vi "flat_Secuence_bloqueo.vi"() -> ()   [LabVIEW 2020]
panel:
  out "Thermometer 4":u8(slide) scale=0.0..100.0
  out "Thermometer 3":u8(slide) scale=0.0..100.0
  out "Thermometer 2":u8(slide) scale=0.0..100.0
  out "Thermometer":u8(slide) scale=0.0..100.0
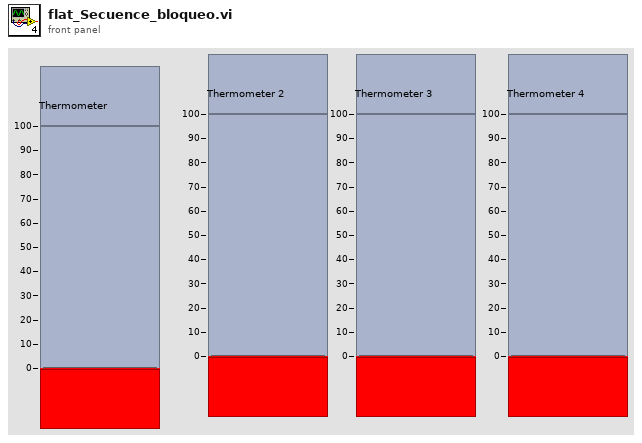
[diagram p1: front panel]
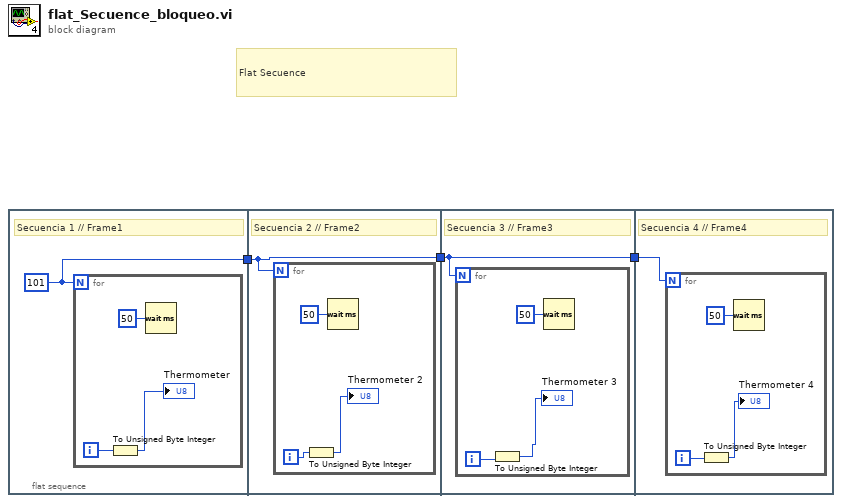
[diagram p0: block diagram]
diagram:
  # "Flat Secuence"
  n1 = flat-sequence {
    tunnel: [w4] -> w3
    tunnel: w3 -> [w8]
    tunnel: [w8] -> w2
    tunnel: w2 -> [w12]
    tunnel: [w12] -> w1
    tunnel: w1 -> [w16]
    frame #0 {
      w4 = 101
      # "Secuencia 1 // Frame1"
      n2 = for {
        N: w4 -> [_]
        i -> [w6]
        n3 = To Unsigned Byte Integer(number=w6) -> (unsigned 8bit integer=→"Thermometer":u8)
        n4 = Wait (ms)(milliseconds to wait=u32 50) -> ()  [unwired: 1 out]
      }
    }
    frame #1 {
      # "Secuencia 2 // Frame2"
      n5 = for {
        N: w8 -> [_]
        i -> [w11]
        n6 = To Unsigned Byte Integer(number=w11) -> (unsigned 8bit integer=→"Thermometer 2":u8)
        n7 = Wait (ms)(milliseconds to wait=u32 50) -> ()  [unwired: 1 out]
      }
    }
    frame #2 {
      # "Secuencia 3 // Frame3"
      n8 = for {
        N: w12 -> [_]
        i -> [w15]
        n9 = To Unsigned Byte Integer(number=w15) -> (unsigned 8bit integer=→"Thermometer 3":u8)
        n10 = Wait (ms)(milliseconds to wait=u32 50) -> ()  [unwired: 1 out]
      }
    }
    frame #3 {
      # "Secuencia 4 // Frame4"
      n11 = for {
        N: w16 -> [_]
        i -> [w19]
        n12 = To Unsigned Byte Integer(number=w19) -> (unsigned 8bit integer=→"Thermometer 4":u8)
        n13 = Wait (ms)(milliseconds to wait=u32 50) -> ()  [unwired: 1 out]
      }
    }
  }
